vi "Handle Last Ack Core.vi"(4 "error in (no error)":errorcluster, 6 "Last Ack":refnum<class "Last Ack.lvclass">, 7 "Caller in":refnum<class "Caller.lvclass">) -> (0 "error out":errorcluster, 3 "Caller out":refnum<class "Caller.lvclass">)   [LabVIEW 2020, in "Caller.lvlib" / "Caller.lvclass"]
doc: "(<B>Filename</B>: Actor Framework.lvlib:Actor.lvclass:Handle Last Ack Core.vi)\n\nDefines how the caller actor responds to the Last Ack message from a nested actor. The Last Ack message is the final message a nested actor sends to its caller before it shuts down. The message contains information about the final state of the nested actor.\n\nBy default, this method does nothing except return any error the nested actor sent. A descendant class may override this method to define behavior."
uses:
  Caller.lvclass
  <vilib>/ActorFramework/LastAck/Last Ack.lvclass
  Caller.lvclass/Caller.ctl
  <vilib>/ActorFramework/Message Enqueuer/Message Enqueuer.lvclass/Message Enqueuer.ctl
  399a52ab-de9c-4f47-9720-846dc4beb769.vi
  399a52ab-de9c-4f47-9720-846dc4beb769.vi/d4db2432-cc9c-482c-8957-dac855435ef6.vi
  399a52ab-de9c-4f47-9720-846dc4beb769.vi/86fbf154-bd7b-49a2-8ab2-a837b2a95f24.vi
  399a52ab-de9c-4f47-9720-846dc4beb769.vi/3b95b01e-1ec2-4565-bcd9-7606a5281010.vi
  399a52ab-de9c-4f47-9720-846dc4beb769.vi/96a08935-737a-44b2-979c-a81d56408f7e.vi
  <vilib>/ActorFramework/Message Enqueuer/Enqueue.vi
  399a52ab-de9c-4f47-9720-846dc4beb769.vi/d4db2432-cc9c-482c-8957-dac855435ef6.vi/6eaecd13-6e48-4772-a921-b51ebdf84d88.vi
  399a52ab-de9c-4f47-9720-846dc4beb769.vi/d4db2432-cc9c-482c-8957-dac855435ef6.vi/d2d5f2b7-06f4-47f6-971c-049c3fdbb653.vi
  399a52ab-de9c-4f47-9720-846dc4beb769.vi/3b95b01e-1ec2-4565-bcd9-7606a5281010.vi/6eaecd13-6e48-4772-a921-b51ebdf84d88.vi
  399a52ab-de9c-4f47-9720-846dc4beb769.vi/3b95b01e-1ec2-4565-bcd9-7606a5281010.vi/d2d5f2b7-06f4-47f6-971c-049c3fdbb653.vi
  399a52ab-de9c-4f47-9720-846dc4beb769.vi/96a08935-737a-44b2-979c-a81d56408f7e.vi/6eaecd13-6e48-4772-a921-b51ebdf84d88.vi
  399a52ab-de9c-4f47-9720-846dc4beb769.vi/96a08935-737a-44b2-979c-a81d56408f7e.vi/d2d5f2b7-06f4-47f6-971c-049c3fdbb653.vi
  Caller Messages/UpdateCPTNested Msg/UpdateCPTNested Msg.lvclass
  C:/Program Files/National Instruments/LabVIEW 2020/vi.lib/ActorFramework/Message/Message.lvclass
  <vilib>/ActorFramework/Message Priority Queue/Priority Enqueue.vi
  <vilib>/ActorFramework/Actor/Actor.lvclass
  <vilib>/Comparison/Less/Less Functor/Less Functor.lvclass
  Nested/Nested.lvclass
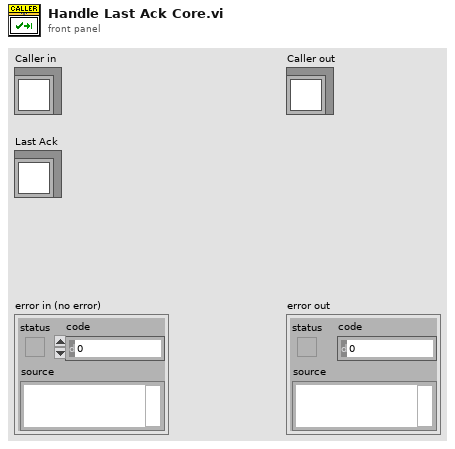
[diagram p1: front panel]
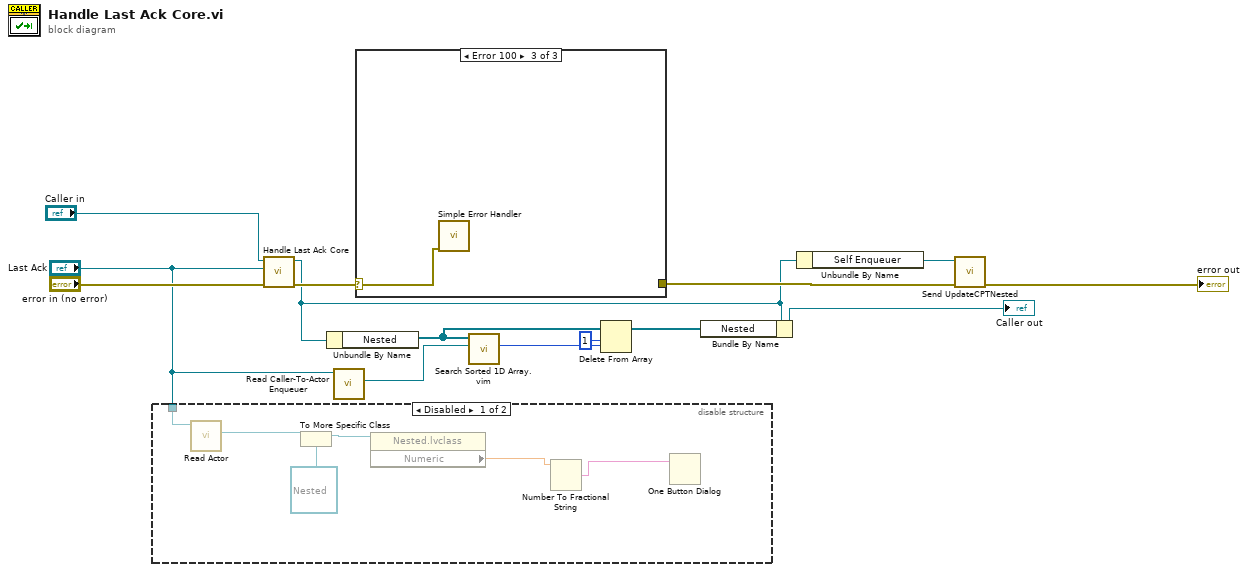
[diagram p0: block diagram]
diagram:
  n1 = disable-structure shown="Disabled" {
    disable-tunnel: "Last Ack" -> [w20 _]
    frame Disabled {
      n2 = call <vilib>:"Read Actor.vi"("Last Ack"=w20) -> ("Actor"=w17:refnum<class "Actor.lvclass">)  [unwired: 10 in]
      n3 = To More Specific Class(target class=refnum<class "Nested.lvclass"> refnum ("Nested.lvlib:Nested.lvclass"), reference=w17) -> (specific class reference=w18:refnum<class "Nested.lvclass">)  [unwired: 1 in, 1 out]
      n4 = property class="Nested.lvclass"(reference=w18) -> ("Numeric"=w16:dbl)  [unwired: 1 in, 2 out]
      n5 = Number To Fractional String(number=w16) -> (F-format string=w15:string)  [unwired: 3 in]
      n6 = One Button Dialog(message=w15) -> ()  [unwired: 1 in, 1 out]
    }
    frame Enabled {
    }
  }
  n7 = call-parent "Handle Last Ack Core.vi"("error in (no error)"="error in (no error)", "Last Ack"="Last Ack", "Actor in"="Caller in") -> ("error out"=w4:errorcluster, "Actor out"=w2:refnum<class "Caller.lvclass">)  [unwired: 3 in]
  n8 = Unbundle By Name(w2) -> ("Nested"=w9:refnum<class "Message Enqueuer.lvclass">[])
  n9 = call <vilib>:"Read Caller-To-Actor Enqueuer.vi"("Last Ack"="Last Ack") -> ("Caller-to-Actor Enqueuer"=w10:refnum<class "Message Enqueuer.lvclass">)  [unwired: 10 in]
  n10 = case shown="Error 100" w4 {
    selector: w4 -> [w21 w22 w23]
    tunnel: [w21 w22 _] -> w3
    frame No Error {
    }
    frame Default {
    }
    frame Error {
      n11 = call <vilib>:"Simple Error Handler.vi"("error in (no error)"=w23) -> ()  [unwired: 4 in, 5 out]
    }
  }
  n12 = call "Search Sorted 1D Array.vim"("element"=w10, "sorted 1D array"=w9) -> ("nearest index"=w8:i32)  [unwired: 8 in, 1 out]
  n13 = Delete From Array(array=w9, length=1, index=w8) -> (array with subset deleted=w5:refnum<class "Message Enqueuer.lvclass">[])  [unwired: 1 out]
  n14 = Bundle By Name(cluster=w2, "Nested"=w5) -> (→"Caller out":refnum<class "Caller.lvclass">)
  n15 = Unbundle By Name(w2) -> ("Self Enqueuer"=w11:refnum<class "Message Enqueuer.lvclass">)
  n16 = call "Send UpdateCPTNested.vi"("error in (no error)"=w3, "Message Enqueuer"=w11) -> ("error out"=→"error out":errorcluster)  [unwired: 8 in, 1 out]
